vi "xeva-setcooling.vi"(8 "error in":errorcluster, 9 "Cooling Set":T1={"iDus"=TRUE, "idus-temp"=-90, "Newton"=TRUE, "newton-temp"=-70, "Clara"=TRUE, "clara-temp"=-55, "Xeva"=TRUE, "xeva-temp"=-70} {"xeva-temp" min=-70 max=20 step=5; "clara-temp" min=-55 max=20 step=5; "newton-temp" min=-90 max=20 step=5; "idus-temp" min=-90 max=20 step=5}, 10 "xeva init":bool caption="xeva-initialized", 11 "xeva-camref":T2) -> (0 "error out":errorcluster, 1 "xenics-status-cluster":T3)   [LabVIEW 2015]
uses:
  <vilib>/Xenics Infrared Solutions/Xeneth LabVIEW API/VIs/Controls/Camara.ctl
  <vilib>/Xenics Infrared Solutions/Xeneth LabVIEW API/Xeneth.lvlib
panel:
  # "Init"
  # "Cooling"
  # "Parameters"
  # "Xeva"
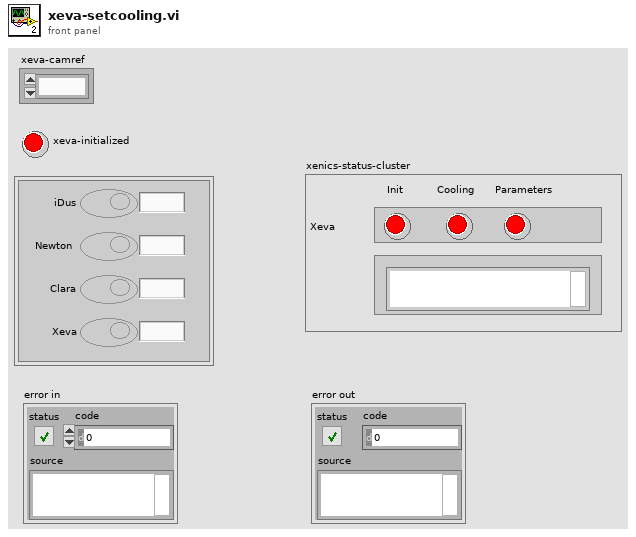
[diagram p1: front panel]
types:
  T1 = cluster{"iDus":bool, "idus-temp":i32, "Newton":bool, "newton-temp":i32, "Clara":bool, "clara-temp":i32, "Xeva":bool, "xeva-temp":i32}
  T2 = typedef "Xeneth.lvlib/Camara.ctl" = refnum<k1>
  T3 = cluster{"Xeva-init":bool, "xeva-cooling":bool, "xeva-parameters":bool, "xeva-error":string}
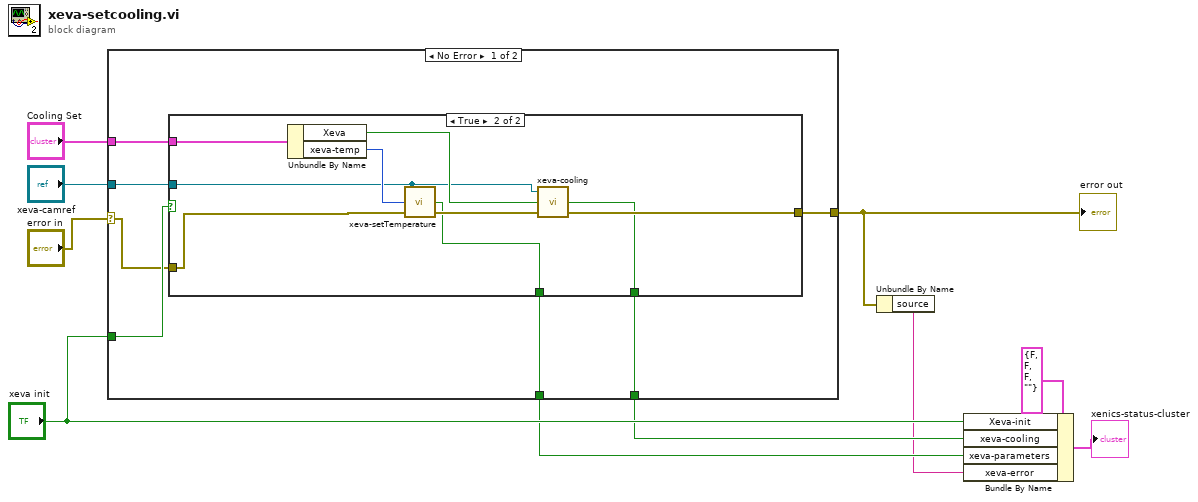
[diagram p0: block diagram]
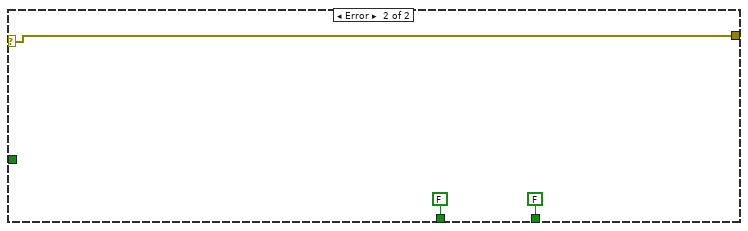
[diagram p3: hidden frame]
diagram:
  n1 = case shown="No Error" "error in" {
    selector: "error in" -> [w11 w31]
    tunnel: "xeva-camref" -> [w17 _]
    tunnel: "Cooling Set" -> [w16 _]
    tunnel: "xeva init" -> [w15 _]
    tunnel: [w14 FALSE ("xeva-temperatureSP-ok")] -> w4
    tunnel: [w13 w31] -> w2
    tunnel: [w12 FALSE ("xeva-cooling")] -> w3
    frame No Error {
      n2 = case shown="True" w15 {
        selector: w15 -> [w19 _]
        tunnel: w17 -> [_ w25]
        tunnel: w16 -> [_ w24]
        tunnel: [w19 w23] -> w14
        tunnel: [w18 w22] -> w13
        tunnel: [w19 w21] -> w12
        tunnel: w11 -> [w18 w20]
        frame False {
        }
        frame True {
          n3 = Unbundle By Name(w24) -> ("Xeva"=w26:bool, "xeva-temp"=w28:i32)
          n4 = call "xeva-setTemperature.vi"("error in (no error)"=w20, "xeva-temperature"=w28, "xeva-camref"=w25) -> ("error out"=w27:errorcluster, "xeva-temperatureSP-ok"=w23:bool)  [unwired: 1 in]
          n5 = call "xeva-cooling.vi"("error in (no error)"=w27, "xeva-cool-on"=w26, "xeva-camref"=w25) -> ("error out"=w22:errorcluster, "xeva-cooling"=w21:bool)  [unwired: 1 in]
        }
      }
    }
    frame Error {
    }
  }
  "error out" <- w2
  n6 = Unbundle By Name(w2) -> ("source"=w1:string)
  n7 = Bundle By Name(cluster=T3 {"Xeva-init"=FALSE, "xeva-cooling"=FALSE, "xeva-parameters"=FALSE, "xeva-error"=""} ("xenics-status-cluster"), "Xeva-init"="xeva init", "xeva-cooling"=w3, "xeva-parameters"=w4, "xeva-error"=w1) -> (→"xenics-status-cluster":T3)
